vi "ble_disconnect_device.vi"(6 "Connection Status":T1={"MAC Address"="", "cnx handle"=0, "cnx flags"=0, "Address Type"=125, "Connection Interval (ms)"=125, "Timeout(ms)"=125, "Latency"=0, "bonding handle"=0} {"Address Type" items=["Public", "Random"]}, 8 "error in (no error)":errorcluster, 11 "COM Bluegiga in":refnum<visa-resource-name>) -> (0 "error out":errorcluster, 3 "COM Bluegiga out":refnum<visa-resource-name>)   [LabVIEW 2017]
uses:
  type_def/connection_status_bundle.ctl
  type_def/address_type.ctl
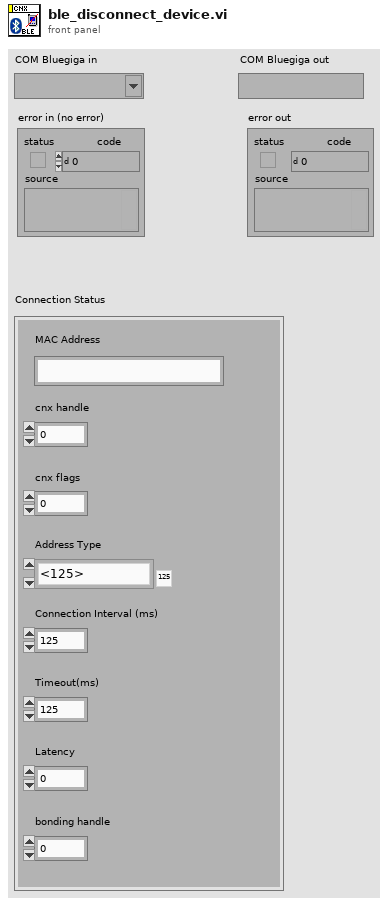
[diagram p1: front panel]
types:
  T1 = typedef "connection_status_bundle.ctl" = cluster{"MAC Address":string, "cnx handle":u8, "cnx flags":u8, "Address Type":T2, "Connection Interval (ms)":u16, "Timeout(ms)":u16, "Latency":u16, "bonding handle":u8}
  T2 = typedef "address_type.ctl" = u8
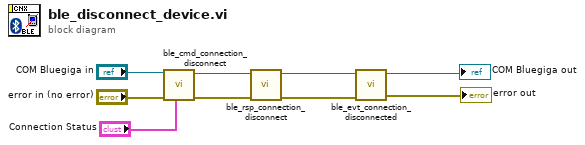
[diagram p0: block diagram]
diagram:
  n1 = call "ble_cmd_connection_disconnect.vi"("Connection Status"="Connection Status", "error in (no error)"="error in (no error)", "COM Bluegiga in"="COM Bluegiga in") -> ("error out"=w5:errorcluster, "COM Bluegiga out"=w6:refnum<visa-resource-name>)  [unwired: 7 in]
  n2 = call "ble_rsp_connection_disconnect.vi"("error in (no error)"=w5, "COM Bluegiga in"=w6) -> ("error out"=w3:errorcluster, "COM Bluegiga out"=w4:refnum<visa-resource-name>)  [unwired: 6 in, 2 out]
  n3 = call "ble_evt_connection_disconnected.vi"("error in (no error)"=w3, "COM Bluegiga in"=w4) -> ("error out"=→"error out":errorcluster, "COM Bluegiga out"=→"COM Bluegiga out":refnum<visa-resource-name>)  [unwired: 8 in]
